vi "GET_operatorID.vi"(8 "error in (no error)":errorcluster, 10 "Operator Full Name":string) -> (0 "error out":errorcluster, 2 "operatorID":u16)   [LabVIEW 2018, in "MySQLTools.lvlib"]
doc: "Take an operator's name as an input and then use the GET_OperatorsTable.vi to return that operatorID as an output."
uses:
  MySQLTools.lvlib
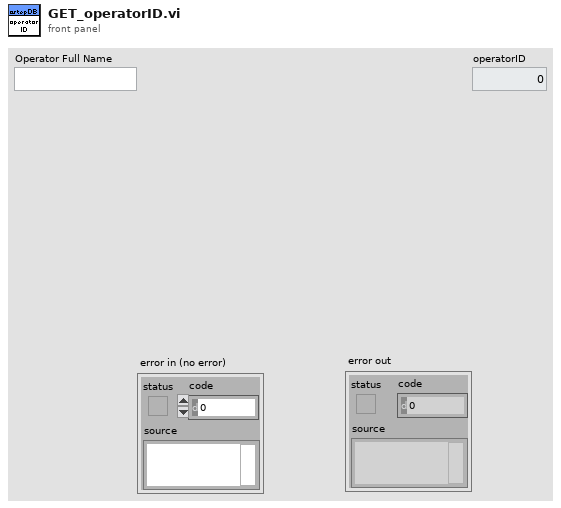
[diagram p1: front panel]
types:
  T1 = typedef "NI_Database_API.lvlib/Conn ObjectReference.ctl" = refnum<k1>
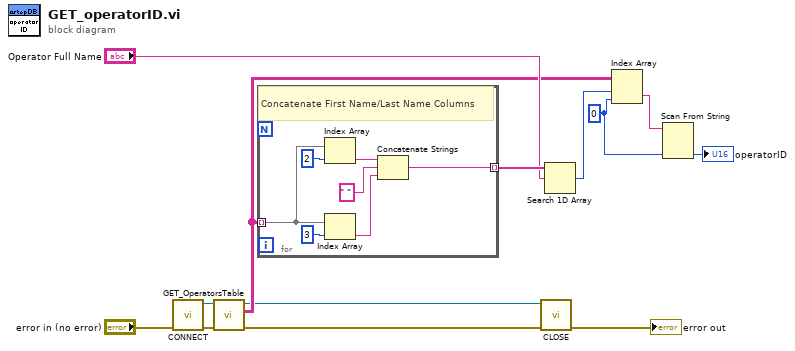
[diagram p0: block diagram]
diagram:
  w8 = u16 0 ("disabled index (col)")
  n1 = call "CONNECT.vi"("error in (no error)"="error in (no error)") -> ("error out"=w2:errorcluster, "connection ref out"=w3:T1)  [unwired: 9 in]
  n2 = call "GET_OperatorsTable.vi"("error in (no error)"=w2, "Database Ref In"=w3) -> ("error out"=w5:errorcluster, "Array"=w10:string[][], "Database Ref Out"=w6:T1)  [unwired: 7 in]
  n3 = for {
    tunnel: w10 -> [w18] mode=indexing
    tunnel: [w14] -> w13 mode=indexing
    # "Concatenate First Name/Last Name Columns"
    n4 = Index Array(array=w18, index=2) -> (element=w16:string)
    n5 = Index Array(array=w18, index=3) -> (element=w17:string)
    n6 = Concatenate Strings(w16, " " ("string"), w17) -> (w14:string)
  }
  n7 = call "CLOSE.vi"("error in (no error)"=w5, "Database Ref In"=w6) -> ("error out"=→"error out":errorcluster)  [unwired: 9 in]
  n8 = Search 1D Array(1D array=w13, element="Operator Full Name") -> (index of element=w11:i32)  [unwired: 1 in]
  n9 = Index Array(array=w10, index (row)=w11, index (col)=w8) -> (element=w9:string)
  n10 = Scan From String(input string=w9, default 1=w8) -> (output 1=→"operatorID":u16)  [unwired: 3 in, 3 out]
